vi "Real Matrix Logarithm_Check Normal.vi"(9 "tolerance":dbl, 10 "Eigenvalues":cdb[](array[numeric]), 11 "Schur Form":T1) -> (3 "normal?":bool)   [LabVIEW 2014, in "NI_AALBase.lvlib"]
uses:
  NI_AALBase.lvlib
  RealMatrix.ctl
  NI_Matrix.lvlib
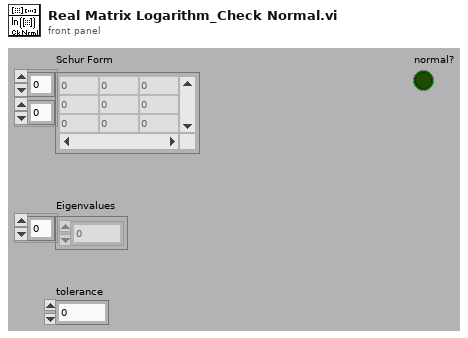
[diagram p1: front panel]
types:
  T1 = typedef "NI_Matrix.lvlib/RealMatrix.ctl" = dbl[][]
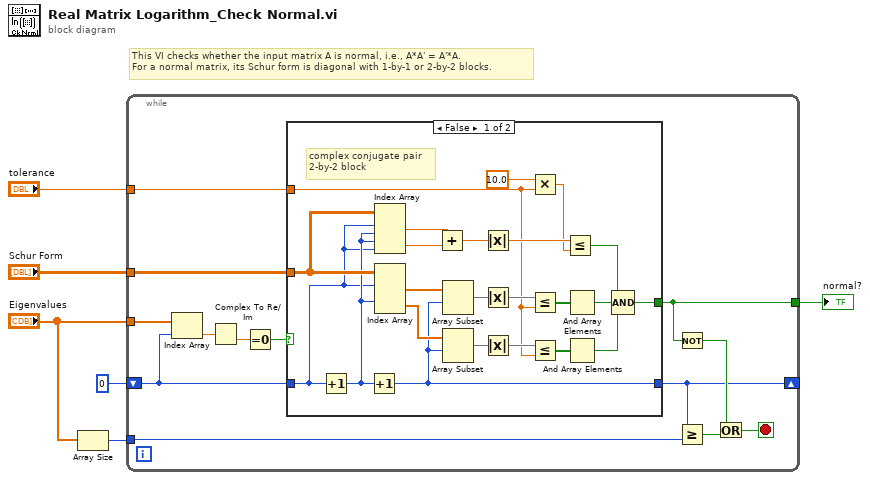
[diagram p0: block diagram]
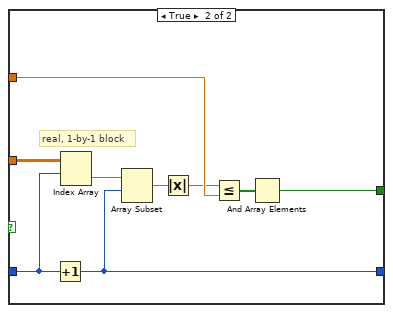
[diagram p2: hidden frame]
diagram:
  # "This VI checks whether the input matrix A is normal, i.e., A*A' = A'*A.\nFor a normal matrix, its Schur form is diagonal with 1-by-1 or 2-by-2 blocks."
  n1 = Array Size(array="Eigenvalues") -> (size(s)=w5:i32)
  n2 = while {
    tunnel: "Eigenvalues" -> [w19]
    tunnel: w5 -> [w15]
    tunnel: "Schur Form" -> [w14]
    tunnel: "tolerance" -> [w13]
    tunnel: [w9] -> w1
    shift-right: [w8] -> _
    shift-left: 0 -> [w7]
    stop <- w10 stop-if-true
    n3 = Index Array(array=w19, index=w7) -> (element=w18:cdb)
    n4 = Complex To Re/Im(x + iy=w18) -> (y=w17:dbl)  [unwired: 1 out]
    n5 = Equal To 0?(x=w17) -> (x = 0?=w16:bool)
    n6 = case shown="False" w16 {
      tunnel: w7 -> [w28 w50]
      tunnel: [w40 w48] -> w8
      tunnel: w14 -> [w30 w51]
      tunnel: w13 -> [w22 w47]
      tunnel: [w33 w44] -> w9
      frame False {
        # "complex conjugate pair\n2-by-2 block"
        n7 = Increment(x=w28) -> (x+1=w29:i32)
        n8 = Increment(x=w29) -> (x+1=w40:i32)
        n9 = Index Array(array=w30, index (row) #1=w28, index (col) #1=w29, index (row) #2=w29, index (col) #2=w28) -> (element #1=w27:dbl, element #2=w26:dbl)
        n10 = Index Array(array=w30, index (row) #1=w28, index (row) #2=w29) -> (element #1=w42:dbl[], element #2=w41:dbl[])  [unwired: 2 in]
        n11 = Add(x=w27, y=w26) -> (x+y=w25:dbl)
        n12 = Array Subset(array=w42, index=w40) -> (w38:dbl[])  [unwired: 1 in]
        n13 = Array Subset(array=w41, index=w40) -> (w36:dbl[])  [unwired: 1 in]
        n14 = Absolute Value(x=w25) -> (abs(x)=w23:dbl)
        n15 = Absolute Value(x=w38) -> (abs(x)=w32:dbl[])
        n16 = Absolute Value(x=w36) -> (abs(x)=w31:dbl[])
        n17 = Multiply(x=10.0, y=w22) -> (x*y=w20:dbl)
        n18 = Less Or Equal?(x=w32, y=w22) -> (x <= y?=w39:bool[])
        n19 = Less Or Equal?(x=w31, y=w22) -> (x <= y?=w37:bool[])
        n20 = Less Or Equal?(x=w23, y=w20) -> (x <= y?=w24:bool)
        n21 = And Array Elements(Boolean array=w39) -> (logical AND=w35:bool)
        n22 = And Array Elements(Boolean array=w37) -> (logical AND=w34:bool)
        n23 = Compound Arithmetic op=AND(w24, w35, w34) -> (w33:bool)
      }
      frame True {
        # "real, 1-by-1 block"
        n24 = Increment(x=w50) -> (x+1=w48:i32)
        n25 = Index Array(array=w51, index (row)=w50) -> (element=w49:dbl[])  [unwired: 1 in]
        n26 = Array Subset(array=w49, index=w48) -> (w46:dbl[])  [unwired: 1 in]
        n27 = Absolute Value(x=w46) -> (abs(x)=w43:dbl[])
        n28 = Less Or Equal?(x=w43, y=w47) -> (x <= y?=w45:bool[])
        n29 = And Array Elements(Boolean array=w45) -> (logical AND=w44:bool)
      }
    }
    n30 = Not(x=w9) -> (.not. x?=w12:bool)
    n31 = Greater Or Equal?(x=w8, y=w15) -> (x >= y?=w11:bool)
    n32 = Or(x=w12, y=w11) -> (x .or. y?=w10:bool)
  }
  "normal?" <- w1
